vi "Average_Reactor_Cool_Loop_ACT_actual_derivative.vi"(0 "SI101_AverageReactorCoolantTemperature.lvclass":refnum<class "SI101.lvclass">, 1 "3 JEC10 CT001B XQ01":dbl, 2 "3 JEC20 CT001B XQ01":dbl, 3 "3 JEC30 CT001B XQ01":dbl, 4 "3 JEC40 CT001B XQ01":dbl, 5 "error in (no error)":errorcluster) -> (14 "SI101_AverageReactorCoolantTemperature.lvclass out":refnum<class "SI101.lvclass">, 15 "ACT 2nd Ctrl":dbl, 16 "ACT D-Comp":dbl, 17 "ACT 2ND MAX LIM":dbl, 19 "error IO":errorcluster)   [LabVIEW 2022 SP3, in "SI101.lvclass"]
uses:
  SI101.lvclass
  SI101.lvclass/SI101.ctl
panel:
  # "SI101"
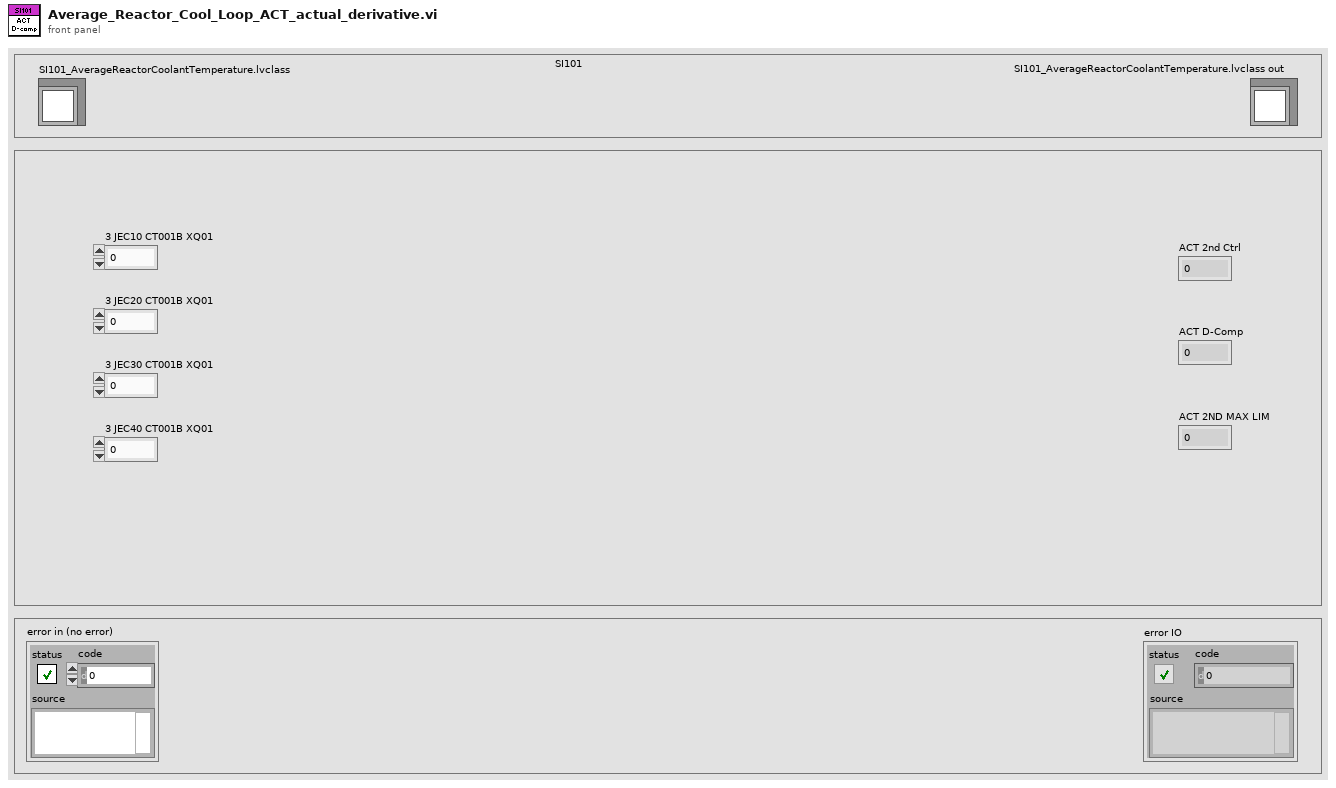
[diagram p1: front panel]
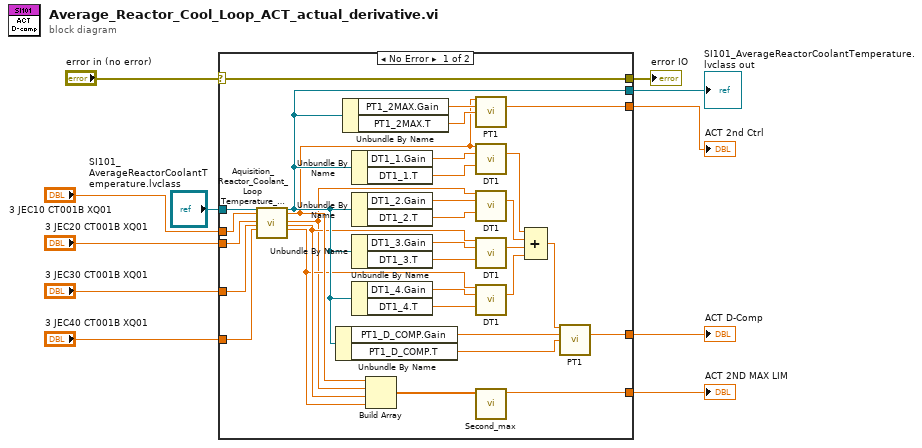
[diagram p0: block diagram]
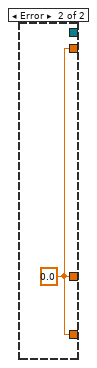
[diagram p2: hidden frame]
diagram:
  n1 = case shown="No Error" "error in (no error)" {
    selector: "error in (no error)" -> [w38 _]
    tunnel: [w39 w44] -> w10
    tunnel: [w24 w44] -> w9
    tunnel: [w38 _] -> w8
    tunnel: [w22 _] -> w7
    tunnel: [w16 w44] -> w6
    tunnel: "SI101_AverageReactorCoolantTemperature.lvclass" -> [w23 _]
    tunnel: "3 JEC10 CT001B XQ01" -> [w15 _]
    tunnel: "3 JEC20 CT001B XQ01" -> [w14 _]
    tunnel: "3 JEC30 CT001B XQ01" -> [w13 _]
    tunnel: "3 JEC40 CT001B XQ01" -> [w12 _]
    frame No Error {
      n2 = call "Aquisition_Reactor_Coolant_Loop Temperature_SG_Inlet_Average.vi"("SI101_AverageReactorCoolantTemperature.lvclass"=w23, "3 JEC10 CT001B XQ01"=w15, "3 JEC20 CT001B XQ01"=w14, "3 JEC30 CT001B XQ01"=w13, "3 JEC40 CT001B XQ01"=w12) -> ("SI101_AverageReactorCoolantTemperature.lvclass out"=w22:refnum<class "SI101.lvclass">, "ACT Loop 1"=w21:dbl, "ACT Loop 2"=w18:dbl, "ACT loop 3"=w20:dbl, "ACT loop 4"=w19:dbl)  [unwired: 17 in, 1 out]
      n3 = Unbundle By Name(w22) -> ("PT1_D_COMP.Gain"=w28:dbl, "PT1_D_COMP.T"=w27:dbl)
      n4 = Unbundle By Name(w22) -> ("PT1_2MAX.Gain"=w26:dbl, "PT1_2MAX.T"=w25:dbl)
      n5 = Unbundle By Name(w22) -> ("DT1_1.Gain"=w36:dbl, "DT1_1.T"=w35:dbl)
      n6 = Unbundle By Name(w22) -> ("DT1_2.Gain"=w34:dbl, "DT1_2.T"=w33:dbl)
      n7 = Unbundle By Name(w22) -> ("DT1_3.Gain"=w32:dbl, "DT1_3.T"=w31:dbl)
      n8 = Unbundle By Name(w22) -> ("DT1_4.Gain"=w30:dbl, "DT1_4.T"=w29:dbl)
      n9 = Build Array(w21, w18, w20, w19) -> (w17:dbl[])
      n10 = call "PT1.vi"("input u(k)"=w21, "G"=w26, "T1"=w25) -> ("output y(k)"=w24:dbl)  [unwired: 11 in, 1 out]
      n11 = call "DT1.vi"("input u(k)"=w21, "G"=w36, "T1"=w35) -> ("output y(k)"=w43:dbl)  [unwired: 11 in, 1 out]
      n12 = call "DT1.vi"("input u(k)"=w18, "G"=w34, "T1"=w33) -> ("output y(k)"=w42:dbl)  [unwired: 11 in, 1 out]
      n13 = call "DT1.vi"("input u(k)"=w20, "G"=w32, "T1"=w31) -> ("output y(k)"=w41:dbl)  [unwired: 11 in, 1 out]
      n14 = call "DT1.vi"("input u(k)"=w19, "G"=w30, "T1"=w29) -> ("output y(k)"=w40:dbl)  [unwired: 11 in, 1 out]
      n15 = call "Second_max.vi"("Array"=w17) -> ("AP3"=w16:dbl)  [unwired: 10 in]
      n16 = Compound Arithmetic op=ADD(w43, w42, w41, w40) -> (w37:dbl)
      n17 = call "PT1.vi"("input u(k)"=w37, "G"=w28, "T1"=w27) -> ("output y(k)"=w39:dbl)  [unwired: 11 in, 1 out]
    }
    frame Error {
      w44 = 0.0 ("output y(k)")
    }
  }
  "ACT D-Comp" <- w10
  "ACT 2nd Ctrl" <- w9
  "SI101_AverageReactorCoolantTemperature.lvclass out" <- w7
  "error IO" <- w8
  "ACT 2ND MAX LIM" <- w6
